vi "MGCC_FntStaMach_Parameter record.vi"   [LabVIEW 2016]
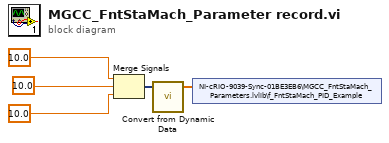
[diagram p0: block diagram]
diagram:
  n1 = Merge Signals(10.0, 10.0, 10.0) -> (w2:dynamicdata)
  n2 = call "Convert from Dynamic Data"("Dynamic Data Type"=w2) -> ("Array"=w1:dbl[])  [unwired: 3 in]
  n3 = shared-variable "NI-cRIO-9039-Sync-01BE3EB6\\MGCC_FntStaMach_Parameters.lvlib\\f_FntStaMach_PID_Example"(w1) -> ()  [unwired: 1 in, 1 out]
